vi "Close GO References (Multiple).vi"(8 "Error In":errorcluster, 11 "References in":refnum<vi>[](array[refnum])) -> (0 "Error Out":errorcluster)   [LabVIEW 2019, in "VI Scripting Tools.lvlib"]
doc: "Use this template to build a VI to use as a subVI."
uses:
  VI Scripting Tools.lvlib
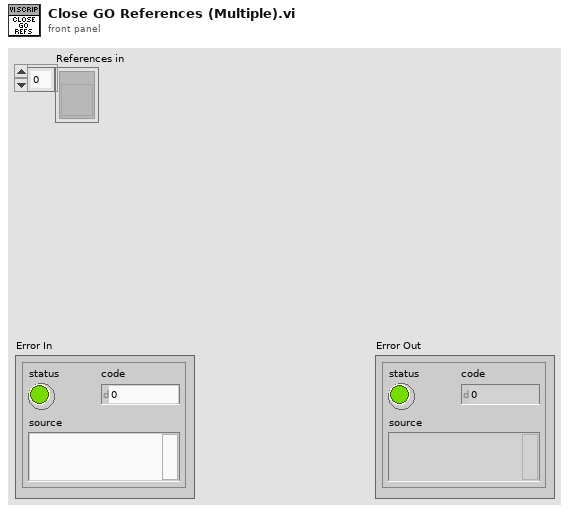
[diagram p1: front panel]
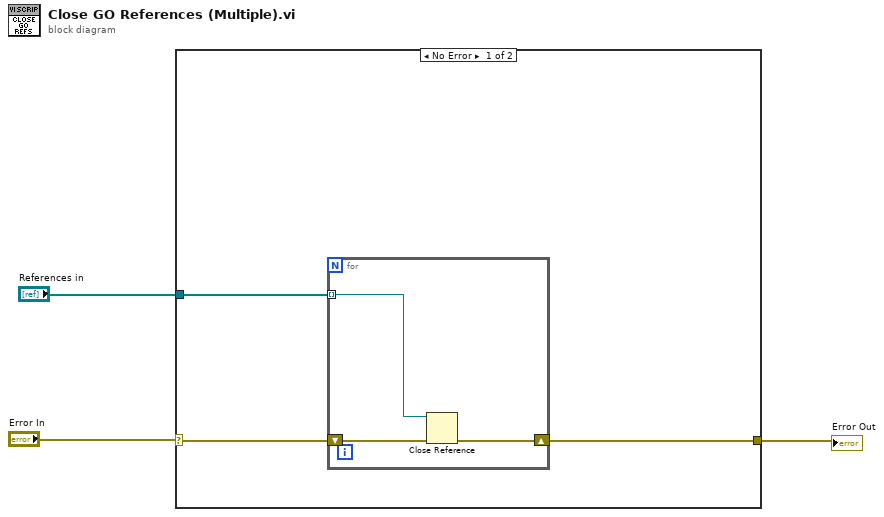
[diagram p0: block diagram]
diagram:
  n1 = case shown="No Error" "Error In" {
    selector: "Error In" -> [w6 w10]
    tunnel: [w5 w10] -> w2
    tunnel: "References in" -> [w4 _]
    frame No Error {
      n2 = for {
        shift-right: [w8] -> w5
        shift-left: w6 -> [w9]
        tunnel: w4 -> [w7] mode=indexing
        n3 = Close Reference(reference=w7, error in (no error)=w9) -> (error out=w8:errorcluster)
      }
    }
    frame Error {
    }
  }
  "Error Out" <- w2
